vi "3.0 Improved Timing Function.vi"(1 "Loop":T1, 2 "Start":u32, 3 "End":u32) -> ()   [LabVIEW 2010]
uses:
  3.0 List of Loops.ctl
  4-High Neurons/4.0-Timing Badass.ctl
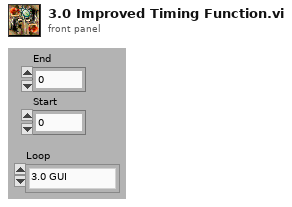
[diagram p1: front panel]
types:
  T1 = typedef "3.0 List of Loops.ctl" = enum16{"3.0 GUI", "3.1 Act", "3.1 4.7.1 Act UDP", "3.1 Joystick", "3.2 Where", "3.2 4.7.2 Where UDP", "3.3 What", "3.3 4.7.3 What UDP", "3.4 How", "3.4 4.7.4 How UDP", "3.5 Limbic", "3.6 Cerebellum"}
  T2 = typedef "4.0-Timing Badass.ctl" = cluster{"Loop Period (ms)":u32, "HB":bool, "Last Time (ms)":u32, "Execution (ms)":u32}
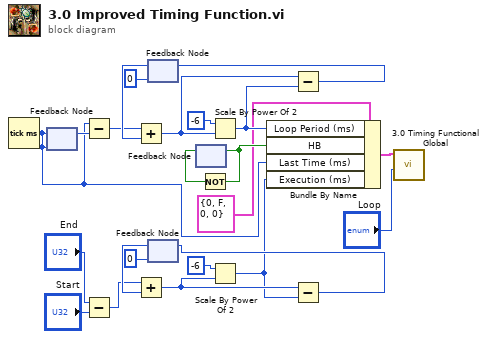
[diagram p0: block diagram]
diagram:
  n1 = Tick Count (ms)() -> (millisecond timer value=w14:u32)
  n2 = feedback #1(w14) -> (w23:u32)
  n3 = feedback-in #1(w14) -> ()
  n4 = Subtract(x=w14, y=w23) -> (x-y=w16:u32)
  n5 = Subtract(x="End", y="Start") -> (x-y=w6:u32)
  n6 = feedback #2(u32 0) -> (w22:u32)
  n7 = Add(x=w16, y=w22) -> (x+y=w21:u32)
  n8 = feedback #3(u32 0) -> (w8:u32)
  n9 = Add(x=w6, y=w8) -> (x+y=w9:u32)
  n10 = feedback #4() -> (w18:bool)  [unwired: 1 in]
  n11 = Not(x=w18) -> (.not. x?=w17:bool)
  n12 = feedback-in #4(w17) -> ()
  n13 = Scale By Power Of 2(n=-6, x=w21) -> (x*2^n=w13:u32)
  n14 = Scale By Power Of 2(n=-6, x=w9) -> (x*2^n=w3:u32)
  n15 = Bundle By Name(cluster=T2 {"Loop Period (ms)"=0, "HB"=FALSE, "Last Time (ms)"=0, "Execution (ms)"=0} ("Loop Update Cluster"), "Loop Period (ms)"=w13, "HB"=w17, "Last Time (ms)"=w14, "Execution (ms)"=w3) -> (w1:T2)
  n16 = Subtract(x=w21, y=w13) -> (x-y=w20:u32)
  n17 = feedback-in #2(w20) -> ()
  n18 = Subtract(x=w9, y=w3) -> (x-y=w7:u32)
  n19 = feedback-in #3(w7) -> ()
  n20 = call "3.0 Timing Functional Global.vi"("Loop"="Loop", "HB In"=w1) -> ()  [unwired: 2 in, 2 out]
